vi "FTW-ActorExtended-Initialize.vi"(0 "FTW Actor Instance Type":refnum<class "FTW-TestStep-Base.lvclass">, 5 "Initialization Job Sequence":string, 7 "Actor Instance Configuration":string, 11 "error in":errorcluster) -> (4 "FTW Actor Instance":refnum<class "FTW-TestStep-Base.lvclass">, 6 "Event Refnums":T1, 15 "error out":errorcluster)   [LabVIEW 2015, in "FTW-TestStep-Base.lvclass"]
uses:
  FTW-TestStep-Base.lvclass
  source/actor/Message/Request/FTW-Message-IncomingRequest.lvclass
  source/actor/Message/Base/FTW-Message.lvclass
  FTW-TestStep-Base.lvclass/FTW-TestStep-Base.ctl
  source/actor/Instance-Extended/FTW-ActorExtended.lvclass
panel:
  # "Inputs"
  # "Outputs"
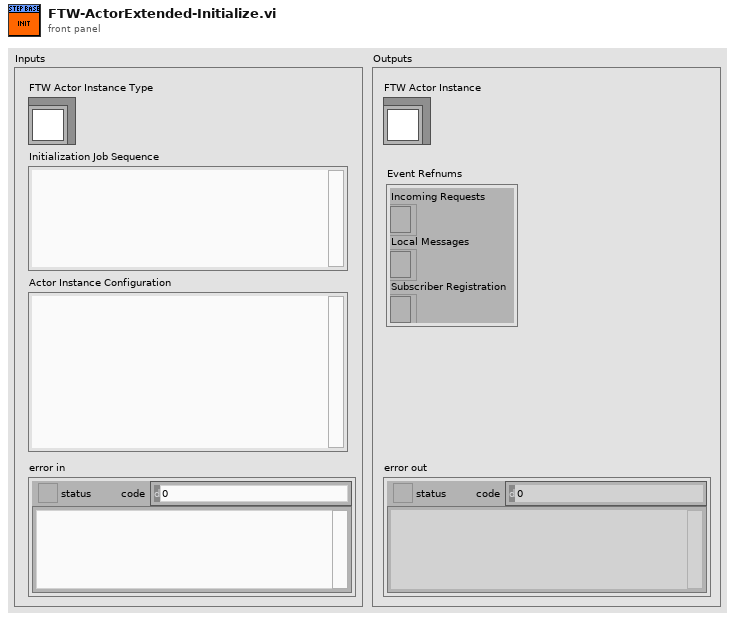
[diagram p1: front panel]
types:
  T1 = cluster{"Incoming Requests":refnum<event-registration>, "Local Messages":refnum<event-registration>, "Subscriber Registration":refnum<event-registration>}
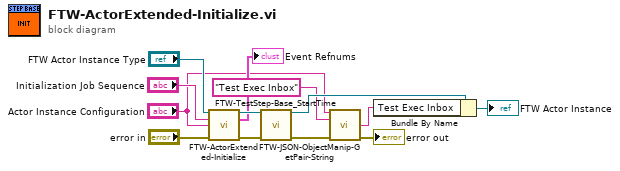
[diagram p0: block diagram]
diagram:
  n1 = call-parent "FTW-ActorExtended-Initialize.vi"("FTW Actor Instance Type"="FTW Actor Instance Type", "Initialization Job Sequence"="Initialization Job Sequence", "Actor Instance Configuration"="Actor Instance Configuration", "error in"="error in") -> ("FTW Actor Instance"=w9:refnum<class "FTW-TestStep-Base.lvclass">, "Event Refnums"=→"Event Refnums":T1, "error out"=w10:errorcluster)  [unwired: 9 in]
  n2 = call-dynamic "FTW-TestStep-Base_StartTime.vi"("FTW-ScripterStep-Base in"=w9, "error in (no error)"=w10) -> ("FTW-ScripterStep-Base out"=w8:refnum<class "FTW-TestStep-Base.lvclass">, "error out"=w5:errorcluster)  [unwired: 12 in]
  n3 = call "FTW-JSON-ObjectManip-GetPair-String.vi"("Input JSON Object"="Actor Instance Configuration", "Key"="Test Exec Inbox", "error in"=w5) -> ("Value"=w1:string, "error out"=→"error out":errorcluster)  [unwired: 9 in, 2 out]
  n4 = Bundle By Name(cluster=w8, "Test Exec Inbox"=w1) -> (→"FTW Actor Instance":refnum<class "FTW-TestStep-Base.lvclass">)
